vi "TESTING W LIMIT SWITCH.vi"() -> ()   [LabVIEW 2019]
uses:
  <vilib>/FPGAPlugInAG/myRIO-1900/niLvFpga_Open_myRIO-1900.vi
  <vilib>/rvi/interface/common/dynamic/niFpgaDynamicAddResources.vi
  <vilib>/Utility/error.llb/Error Cluster From Error Code.vi
  <vilib>/rvi/errors/niLvFpgaAdjustHostInterfaceError.vi
  <vilib>/rvi/interface/nirviOpenFPGA/nirviOpenFPGA.xnode
  Collin's Project/FPGA Bitfiles/MRmecanum_FPGATarget_FPGAMainModified_TerasRobot_LKSN2021.lvbitx
  <vilib>/rvi/interface/nirviReadWriteControl/nirviReadWriteControl.xnode
  <vilib>/rvi/interface/Simulation/niFpgaSimulationCallBeginRW.vi
  NiFpgaLv.dll
panel:
  out "LIMIT SWITCH 1":bool
  out "START BUTTON":bool
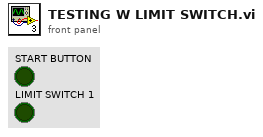
[diagram p1: front panel]
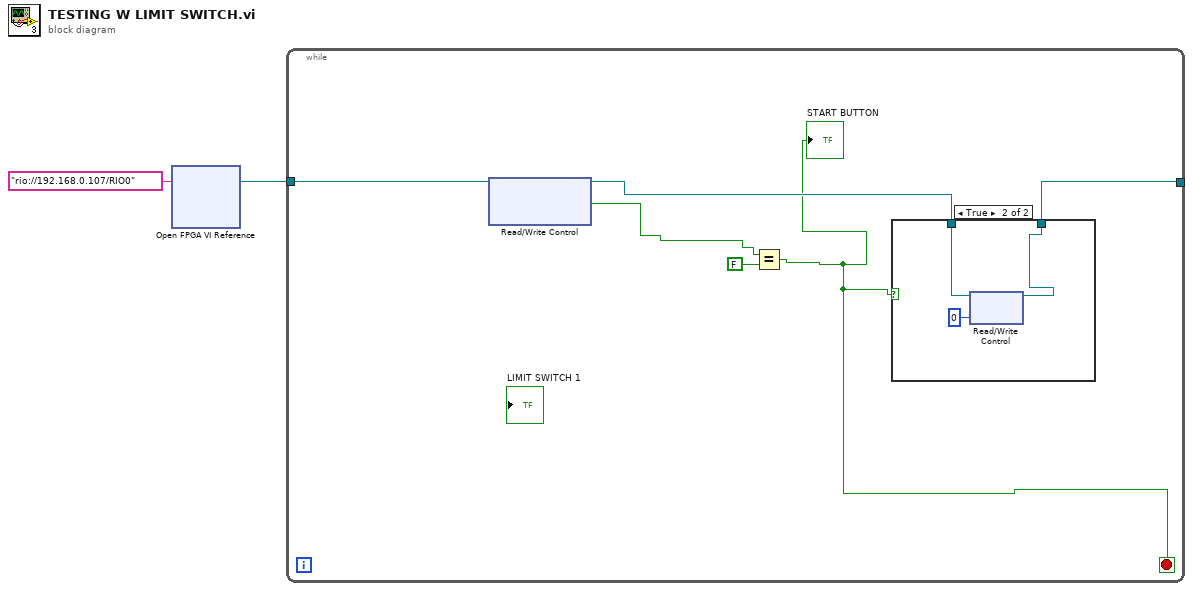
[diagram p0: block diagram]
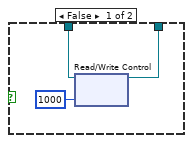
[diagram p2: hidden frame]
diagram:
  n1 = xnode "Open FPGA VI Reference"("resource name"=tag "rio://192.168.0.107/RIO0") -> ("FPGA VI Reference Out"=w1:refnum<k20>)  [unwired: 1 in, 1 out]
  n2 = while {
    tunnel: w1 -> [w8]
    tunnel: [w6] -> _
    stop <- w3 stop-if-true
    n3 = xnode "Read/Write Control"("FPGA VI Reference In"=w8) -> ("FPGA VI Reference Out"=w7:refnum<k20>, "START BUTTON"=w5:bool)  [unwired: 1 in, 2 out]
    n4 = Equal?(x=w5, y=FALSE) -> (x = y?=w3:bool)
    "START BUTTON" <- w3
    n5 = case shown="True" w3 {
      tunnel: w7 -> [w11 w14]
      tunnel: [w10 w13] -> w6
      frame False {
        n6 = xnode "Read/Write Control"("FPGA VI Reference In"=w11, "M4"=i16 1000) -> ("FPGA VI Reference Out"=w10:refnum<k20>)  [unwired: 1 in, 1 out]
      }
      frame True {
        n7 = xnode "Read/Write Control"("FPGA VI Reference In"=w14, "M4"=i16 0) -> ("FPGA VI Reference Out"=w13:refnum<k20>)  [unwired: 1 in, 1 out]
      }
    }
  }
